vi "App Path.vi"() -> (2 "App Path":path)   [LabVIEW 2020, in "Volatus.lvlib"]
uses:
  Volatus.lvlib
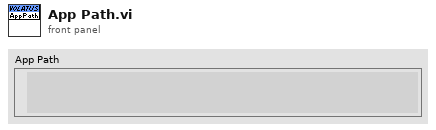
[diagram p1: front panel]
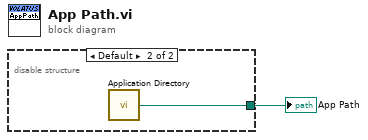
[diagram p0: block diagram]
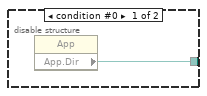
[diagram p2: hidden frame]
diagram:
  n1 = disable-structure shown="Default" {
    disable-tunnel: [w2 w3] -> w1
    frame condition #0 {
      n2 = property class="App"() -> ("App.Dir"=w2:path)  [unwired: 2 in, 2 out]
    }
    frame condition #1 (active) {
      n3 = call <vilib>:"Application Directory.vi"() -> ("Application Directory"=w3:path)
    }
  }
  "App Path" <- w1
